vi "GETwithRetry.vi"(8 "error in (no error)":errorcluster, 9 "request specific headers":T1[](array[typedef]), 10 "String":string, 11 "REST Client in":refnum<class "REST Client.lvclass">) -> (0 "error out":errorcluster, 1 "Response body":string, 2 "Status String":string, 3 "REST Client out":refnum<class "REST Client.lvclass">)   [LabVIEW 2024]
uses:
  <vilib>/addons/_JKI.lib/REST Client/classes/REST Client/REST Client.lvclass
  <vilib>/addons/_JKI.lib/REST Client/classes/REST Client/HTTP Header.ctl
  <vilib>/NI/Advanced HTTP Client/Header--Combo Box.ctl
  <vilib>/NI/Advanced HTTP Client/Session.lvclass
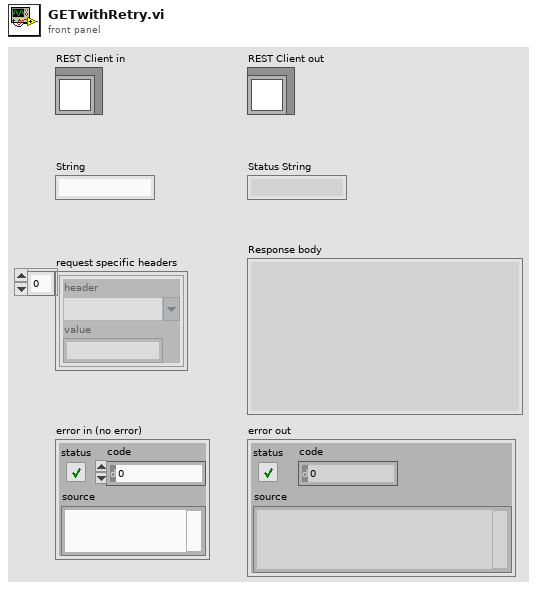
[diagram p1: front panel]
types:
  T1 = typedef "REST Client.lvlib/REST Client.lvclass/HTTP Header.ctl" = cluster{"header":T2, "value":string}
  T2 = typedef "lib_NI_Advanced HTTP Client.lvlib/Session.lvclass/Header--Combo Box.ctl" = string
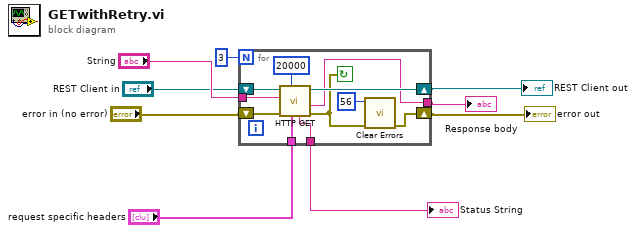
[diagram p0: block diagram]
diagram:
  n1 = for {
    N: 3 -> [_]
    shift-right: [w18] -> w8
    shift-left: "REST Client in" -> [w19]
    shift-right: [w14] -> w9
    shift-left: "error in (no error)" -> [w20]
    tunnel: "String" -> [w13]
    tunnel: [w12] -> w1
    tunnel: "request specific headers" -> [w11]
    tunnel: [w10] -> w6
    stop <- w15 continue-if-true
    n2 = call-dynamic "HTTP GET.vi"("request specific headers"=w11, "timeout (0 = Use Default)"=20000, "error in (no error)"=w20, "Path"=w13, "REST Client in"=w19) -> ("error out"=w15:errorcluster, "Response body"=w12:string, "REST Client out"=w18:refnum<class "REST Client.lvclass">, "Status String"=w10:string)  [unwired: 1 in, 2 out]
    n3 = call <vilib>:"Clear Errors.vi"("error in (no error)"=w15, "specific error code to clear (0: all)"=56) -> ("error out"=w14:errorcluster)  [unwired: 4 in, 1 out]
  }
  "error out" <- w9
  "REST Client out" <- w8
  "Status String" <- w6
  "Response body" <- w1
